vi "Offset_Gain_new.vi"() -> ()   [LabVIEW 2019]
uses:
  <userlib>/_TI-LA/Instr Drivers/Signal Generator/33XXX/Driver/EasyIO/Typedef/33XXX Standard Waveform Configuration.ctl
  <userlib>/_TI-LA/Instr Drivers/Signal Generator/33XXX/Driver/EasyIO/Typedef/33XXX Waveform Function.ctl
  <userlib>/_TI-LA/Instr Drivers/Signal Generator/33XXX/Driver/EasyIO/Typedef/33XXX Waveform Unit.ctl
  <userlib>/_TI-LA/Instr Drivers/Signal Generator/33XXX/Driver/EasyIO/Typedef/33XXX Output Load.ctl
  <userlib>/_TI-LA/Instr Drivers/Signal Generator/33XXX/Driver/EasyIO/Typedef/33XXX Output Load Termination.ctl
  <instrlib>/Agilent 34401/Public/Data/Read (Single Point).vi
  <userlib>/_TI-LA/Instr Drivers/Signal Generator/33XXX/Modules/33XXX Modules.lvlib
  <userlib>/_TI-LA/Instr Drivers/Signal Generator/33XXX/Driver/33XXX.lvlib
  <vilib>/Analysis/NI_AALPro.lvlib
  <instrlib>/Agilent 34401/Agilent 34401.lvlib
  <vilib>/Utility/file.llb/Write Delimited Spreadsheet (DBL).vi
panel:
  out "Measured Input":dbl[](array[numeric])
  out "Measured Vref":dbl
  out "Gain Error (LSB)":dbl
  out "Offset Error (mV)":dbl
  out "slope":dbl
  out "intercept":dbl
  out "Measure Codes":dbl[](array[numeric])
  in  "lv_scomp":u16=8
  in  "lv_ref_vol":u16
  in  "lv_ref_sel":u16
  in  "Standard Waveform Configuration":T1={"Frequency (Hz)"=1000.0, "Waveform Function"=1, "DC Offset (V)"=0.0, "Unit"=0, "Amplitude (V)"=1.0, "Duty cycle (%)"=50.0} {"Duty cycle (%)" min=0.002 max=99.999 step=0.001 format="%.3p"; "Amplitude (V)" min=0.001 max=20.0 format="%#_6p"; "Unit" items=["Vpp", "Vrms", "dB"]; "DC Offset (V)" min=-10.0 max=10.0 format="%#_6p"; "Waveform Function" items=["DC", "Sine", "Square", "Triangle", "Ramp", "Pulse", "Noise", "Sinc", "Negative Ramp", "Exponential Rise", "Exponential Fall", "Cardiac"]; "Frequency (Hz)" min=1e-06 max=80000000.0 format="%#_6p"}
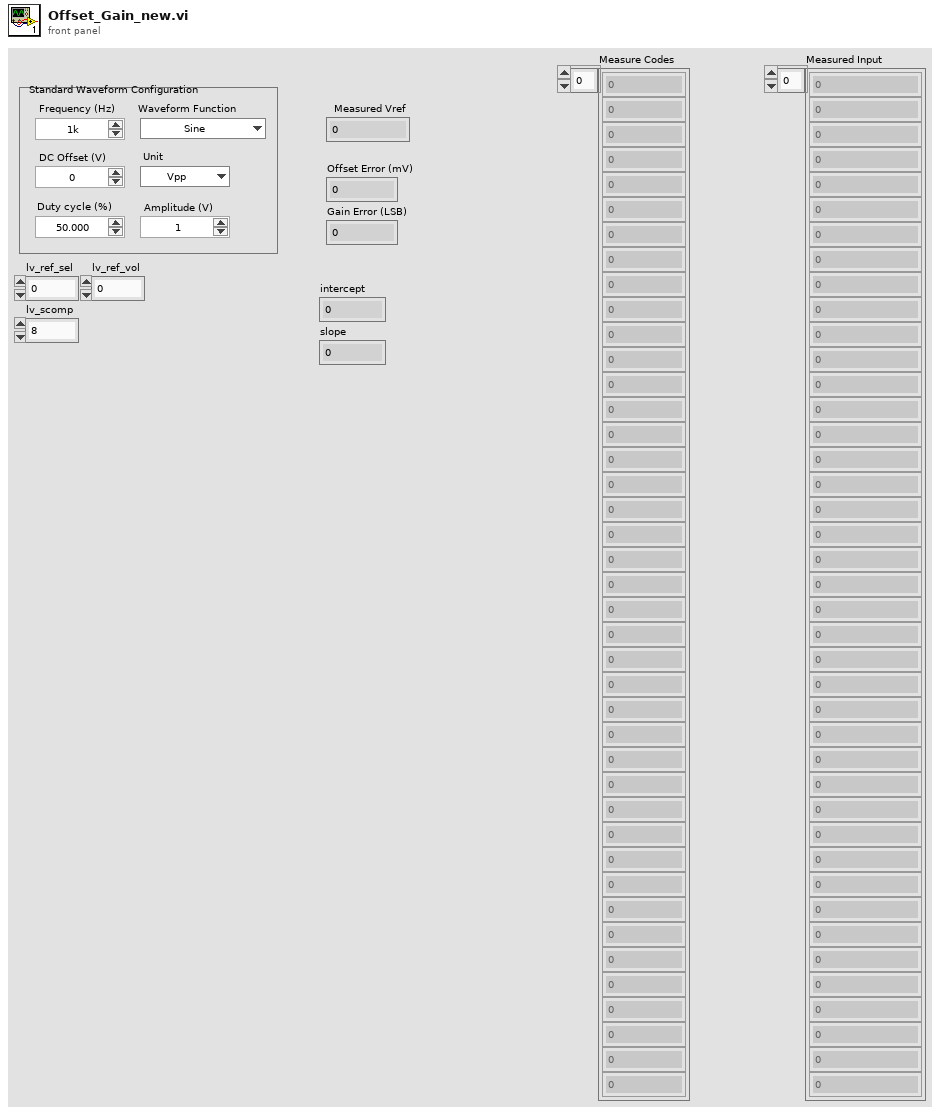
[diagram p1: front panel]
types:
  T1 = typedef "33XXX.lvlib/33XXX Standard Waveform Configuration.ctl" = cluster{"Frequency (Hz)":dbl, "Waveform Function":T2, "DC Offset (V)":dbl, "Unit":T3, "Amplitude (V)":dbl, "Duty cycle (%)":dbl}
  T2 = typedef "33XXX.lvlib/33XXX Waveform Function.ctl" = u16
  T3 = typedef "33XXX.lvlib/33XXX Waveform Unit.ctl" = u16
  T4 = typedef "33XXX.lvlib/33XXX Output Load.ctl" = cluster{"Output Load Impedence":T5, "Load value (ohms)":dbl}
  T5 = typedef "33XXX.lvlib/33XXX Output Load Termination.ctl" = enum16{"50 Ohms", "High Z", "User Defined"}
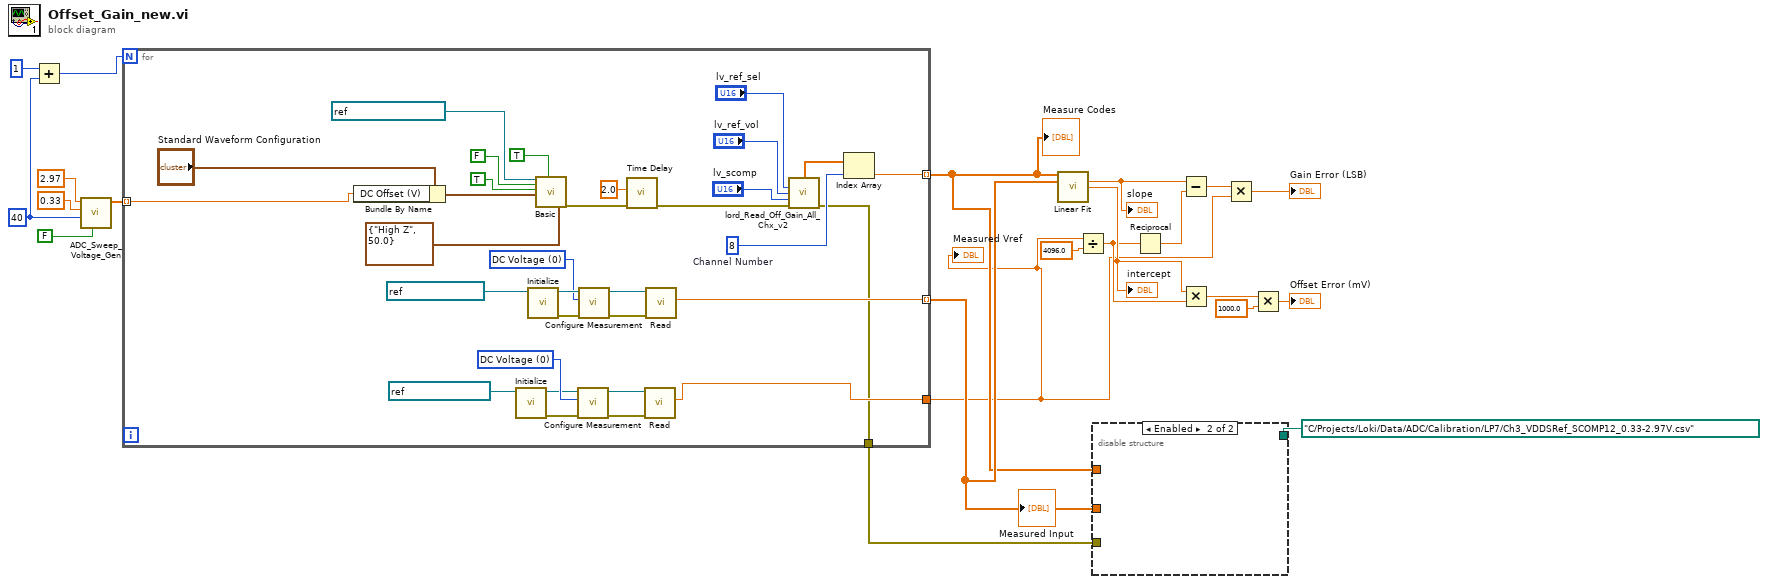
[diagram p0: block diagram]
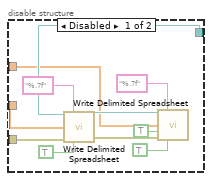
[diagram p2: hidden frame]
diagram:
  w7 = 40 ("Count")
  n1 = Add(x=1, y=w7) -> (x+y=w8:i32)
  n2 = call "ADC_Sweep_Voltage_Gen.vi"("Shuffle"=FALSE, "Count"=w7, "Vn"=0.33, "Vp"=2.97) -> ("Vin_Array_Set"=w19:dbl[])  [unwired: 7 in]
  n3 = for {
    N: w8 -> [_]
    tunnel: w19 -> [w30] mode=indexing
    tunnel: [w49] -> w2 mode=indexing
    tunnel: [w25] -> w5 mode=indexing
    tunnel: [w24] -> w1
    tunnel: [w23] -> w3
    w29 = u16 0 items=["DC Voltage", "AC Voltage", "2 - Wire Resistance", "4 - Wire Resistance", "DC Current", "AC Current", "Frequency", "Period", "Continuity", "Diode Checking", "VDC:VDC Ratio", "Temperature", "Capacitance"] ("Function (0: DC Voltage)")
    w38 = u16 0 items=["DC Voltage", "AC Voltage", "2 - Wire Resistance", "4 - Wire Resistance", "DC Current", "AC Current", "Frequency", "Period", "Continuity", "Diode Checking", "VDC:VDC Ratio", "Temperature", "Capacitance"] ("Function (0: DC Voltage)")
    w50 = 8  # Channel Number
    n4 = Bundle By Name(cluster="Standard Waveform Configuration", "DC Offset (V)"=w30) -> (w53:T1)
    n5 = call <instrlib>:"Initialize.vi"("VISA resource name"=refnum<visa-resource-name> "GPIB0::5::INSTR") -> ("error out"=w40:errorcluster, "VISA resource name out"=w37:refnum<visa-resource-name>)  [unwired: 9 in]
    n6 = call <instrlib>:"Initialize.vi"("VISA resource name"=refnum<visa-resource-name> "GPIB0::6::INSTR") -> ("error out"=w33:errorcluster, "VISA resource name out"=w34:refnum<visa-resource-name>)  [unwired: 9 in]
    n7 = call <userlib>:"Basic.vi"("Instrument Address"=refnum<visa-resource-name> "GPIB0::10::INSTR", "Reset?"=FALSE, "ID Query?"=TRUE, "Standard Waveform Configuration"=w53, "Enable Output?"=TRUE, "Output Load Configuration"=T4 {"Output Load Impedence"=enum."High Z", "Load value (ohms)"=50.0}) -> ("error out"=w27:errorcluster)  [unwired: 11 in, 2 out]
    n8 = call <instrlib>:"Configure Measurement.vi"("error in (no error)"=w40, "Function (0: DC Voltage)"=w38, "VISA resource name"=w37) -> ("error out"=w39:errorcluster, "VISA resource name out"=w36:refnum<visa-resource-name>)  [unwired: 7 in]
    n9 = call <instrlib>:"Configure Measurement.vi"("error in (no error)"=w33, "Function (0: DC Voltage)"=w29, "VISA resource name"=w34) -> ("error out"=w32:errorcluster, "VISA resource name out"=w31:refnum<visa-resource-name>)  [unwired: 7 in]
    n10 = call "Time Delay"("error in (no error)"=w27, "Delay Time (s)"=2.0) -> ("error out"=w45:errorcluster)  [unwired: 9 in]
    n11 = call-poly <instrlib>:"Read.vi"("error in (no error)"=w39, "VISA resource name"=w36) -> ("Measurement"=w24:dbl)  [unwired: 7 in, 2 out]
    n12 = call-poly <instrlib>:"Read.vi"("error in (no error)"=w32, "VISA resource name"=w31) -> ("Measurement"=w25:dbl)  [unwired: 7 in, 2 out]
    n13 = call "lord_Read_Off_Gain_All_Chx_v2.vi"("lv_ref_sel"="lv_ref_sel", "lv_ref_vol"="lv_ref_vol", "lv_scomp"="lv_scomp", "error in"=w45) -> ("Mean[]"=w51:dbl[], "error out"=w23:errorcluster)  [unwired: 3 in, 7 out]
    n14 = Index Array(array=w51, index=w50) -> (element=w49:dbl)
  }
  "Measure Codes" <- w2
  "Measured Vref" <- w1
  "Measured Input" <- w5
  n15 = call <vilib>:"Linear Fit.vi"("Y"=w2, "X"=w5) -> ("slope"=w14:dbl, "intercept"=w18:dbl)  [unwired: 9 in, 3 out]
  "intercept" <- w18
  "slope" <- w14
  n16 = Divide(x=w1, y=4096.0) -> (x/y=w10:dbl)
  n17 = disable-structure shown="Enabled" {
    disable-tunnel: w5 -> [w65 _]
    disable-tunnel: path "C:/Projects/Loki/Data/ADC/Calibration/LP7/Ch3_VDDSRef_SCOMP12_0.33-2.97V.csv" ("file path (dialog if empty)") -> [w64 _]
    disable-tunnel: w3 -> [w63 _]
    disable-tunnel: w2 -> [w60 _]
    frame Disabled {
      n18 = call-poly <vilib>:"Write Delimited Spreadsheet.vi"("file path (dialog if empty)"=w64, "format (%.3f)"="%.7f", "1D data"=w65, "error in (no error)"=w63, "transpose? (no:F)"=TRUE) -> ("new file path (Not A Path if cancelled)"=w61:path, "error out"=w59:errorcluster)  [unwired: 9 in]
      n19 = call-poly <vilib>:"Write Delimited Spreadsheet.vi"("file path (dialog if empty)"=w61, "format (%.3f)"="%.7f", "1D data"=w60, "append to file? (new file:F)"=TRUE, "error in (no error)"=w59, "transpose? (no:F)"=TRUE) -> ()  [unwired: 8 in, 2 out]
    }
    frame Enabled {
    }
  }
  n20 = Reciprocal(x=w10) -> (1/x=w9:dbl)
  n21 = Subtract(x=w14, y=w9) -> (x-y=w13:dbl)
  n22 = Multiply(x=w18, y=w10) -> (x*y=w16:dbl)
  n23 = Multiply(x=w13, y=w1) -> (x*y=→"Gain Error (LSB)":dbl)
  n24 = Multiply(x=w16, y=1000.0) -> (x*y=→"Offset Error (mV)":dbl)
